vi "Main NR.vi"(8 "error in":errorcluster, 11 "cRIO NI 9205 Demo in":refnum<class "cRIO NI 9205 Demo.lvclass">) -> (0 "error out":errorcluster, 3 "cRIO NI 9205 Demo out":refnum<class "cRIO NI 9205 Demo.lvclass">)   [LabVIEW 2017, in "cRIO NI 9205 Demo.lvclass"]
doc: "The <b>Queued Message Handler</b> of the Worker that owns this VI."
uses:
  cRIO NI 9205 Demo.lvclass
  C:/Program Files (x86)/National Instruments/LabVIEW 2017/vi.lib/addons/_Workers/Library/Classes/Worker/Worker.lvclass
  cRIO NI 9205 Demo.lvclass/cRIO NI 9205 Demo.ctl
  Initialization Data.ctl
  TCP Client/TCP Client/rwr_Connect to Server.ctl
  Shared/TCP Data KEYS.ctl
  Shared/TCP Data Format.ctl
  TCP Client/TCP Client/rqp_Send String to Server.ctl
  <vilib>/addons/_Workers/Library/Classes/Message Queue/Message Queue.lvclass
  RT System Monitor/RT System Monitor.lvclass
  FPGA Read/FPGA Read.lvclass
  RT Watchdog/RT Watchdog.lvclass
  TCP Client/TCP Client/TCP Client.lvclass
panel:
  out "IP Address":string caption="Server IP Address"
  out "Server name":string caption="Server Name"
  out "Connected?":bool
  # "Server Connected"
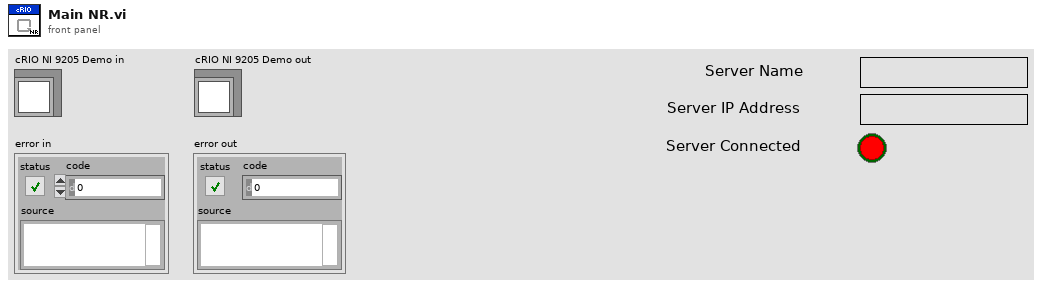
[diagram p1: front panel]
types:
  T1 = typedef "cRIO NI 9205 Demo.lvclass/Initialization Data.ctl" = cluster{"Client Name":string, "Server IP Address":string, "Server Port":u16, "Debugging Mode?":bool}
  T2 = typedef "TCP Client.lvlib/TCP Client.lvclass/rwr_Connect to Server.ctl" = cluster{"Client Name":string, "Server IP Address":string, "Server Port":u16}
  T3 = typedef "TCP Client.lvlib/TCP Client.lvclass/rqp_Send String to Server.ctl" = cluster{"String to Send":string}
  T4 = typedef "TCP Data Format.ctl" = cluster{"KEY":T5, "Data":string}
  T5 = typedef "TCP Data KEYS.ctl" = enum16{"RT System Monitor", "FPGA Data"}
  T6 = typedef "TCP Client.lvlib/TCP Client.lvclass/rsp_Connection Notify.ctl" = cluster{"Server Name":string, "IP Address":string, "Connected?":bool}
  T7 = typedef "RT System Monitor.lvclass/rsp_Receive System Properties.ctl" = cluster{"System Health Data":T8}
  T8 = typedef "System Health Data.ctl" = cluster{"CPUs":u32[][], "Memory":dbl[][], "Hard Drive Space Used (%)":dbl, "Primary Hard Drive Available (MB)":dbl, "Primary Hard Drive Capacity (MB)":u32, "Total Physical Memory (MB)":u32, "Total Virtual Memory (MB)":u32}
  T9 = typedef "FPGA Read.lvclass/rsp_Receive FPGA Data.ctl" = cluster{"FPGA Data":fxp<+/-,26,5>[]}
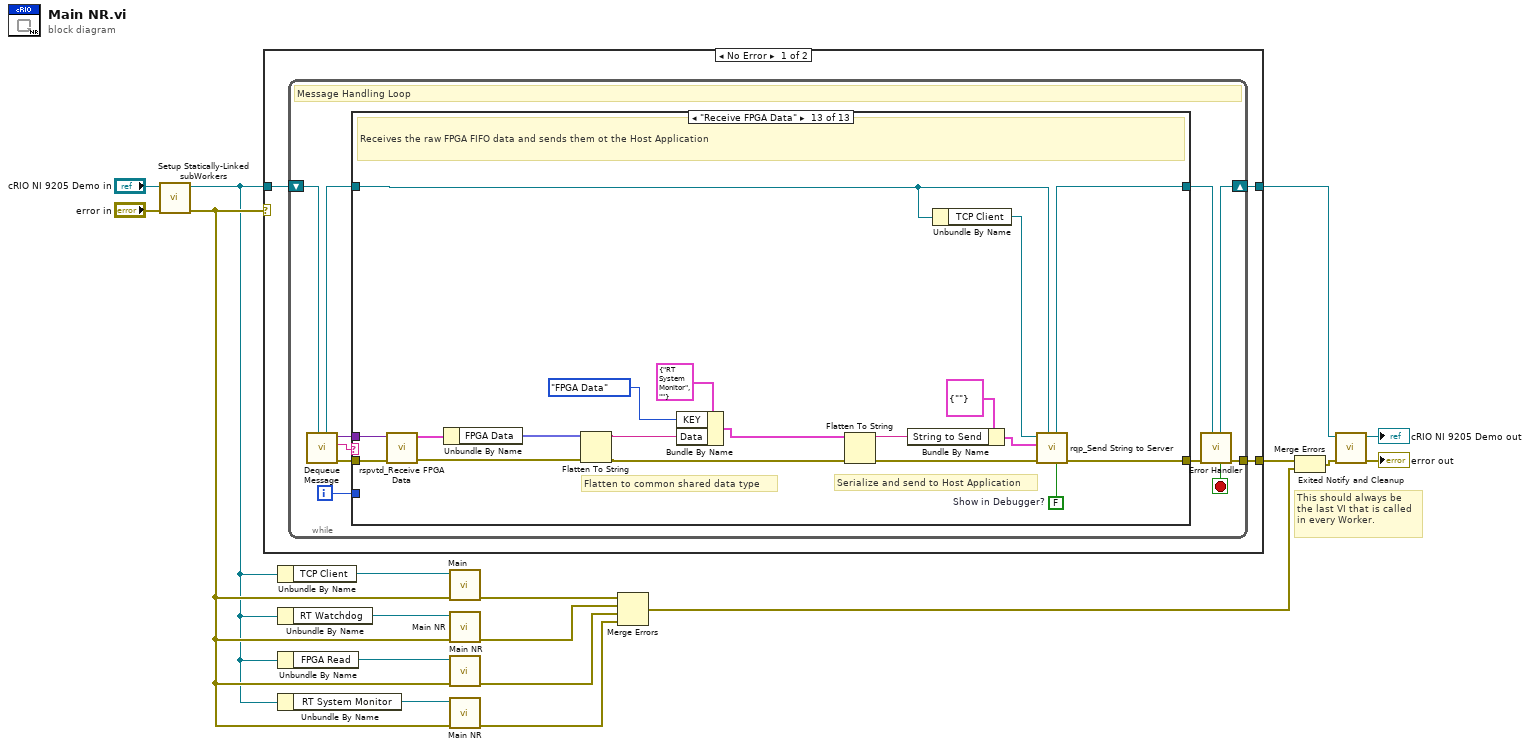
[diagram p0: block diagram]
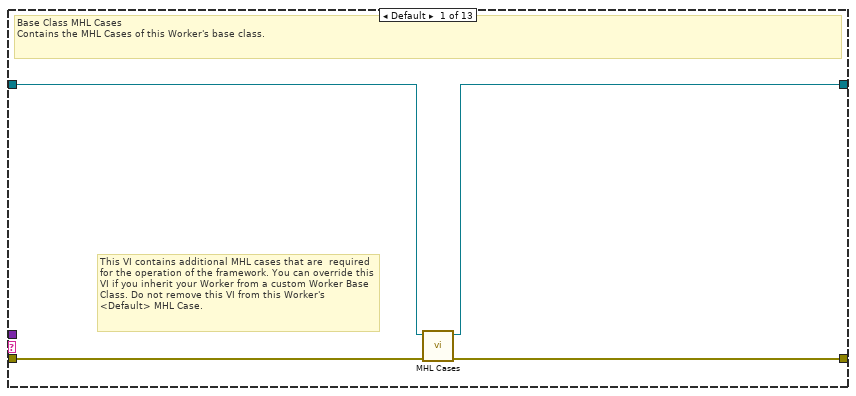
[diagram p2: hidden frame]
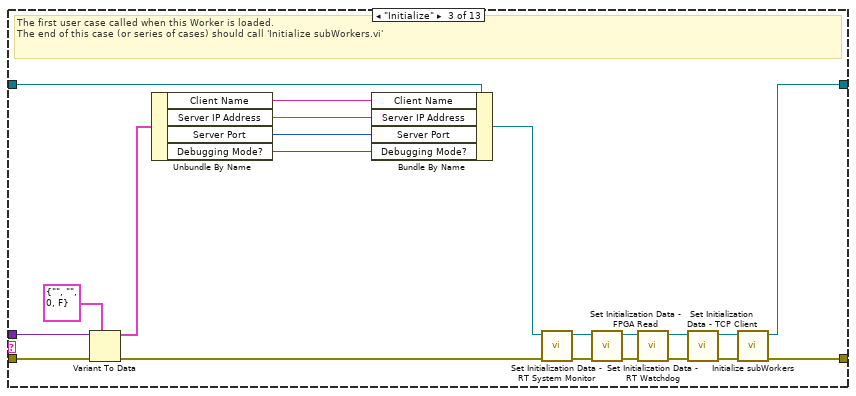
[diagram p4: hidden frame]
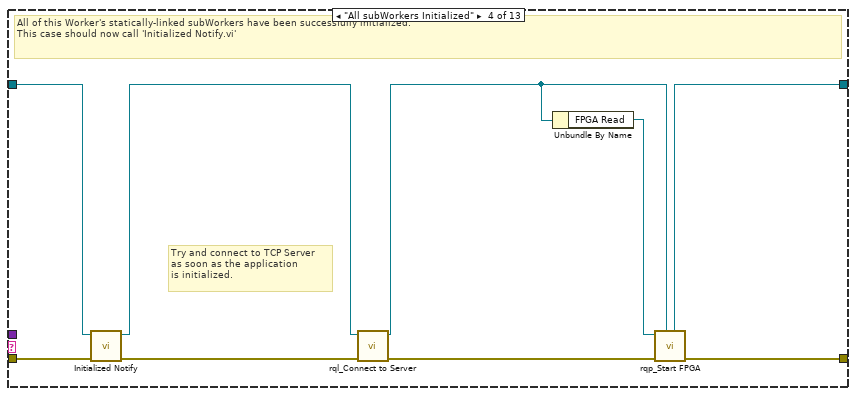
[diagram p5: hidden frame]
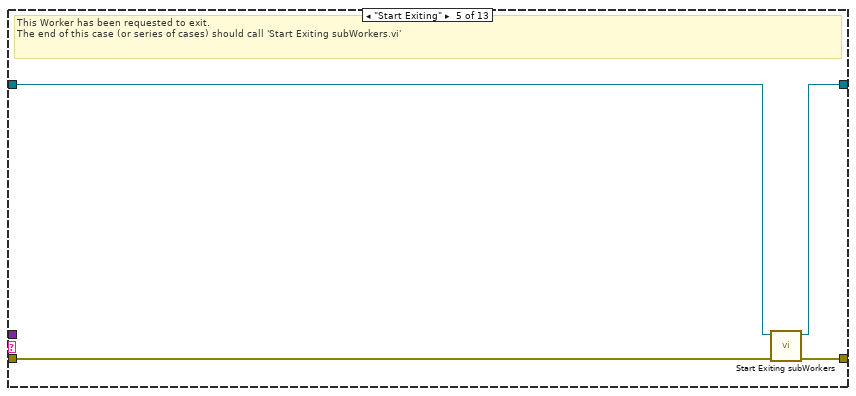
[diagram p6: hidden frame]
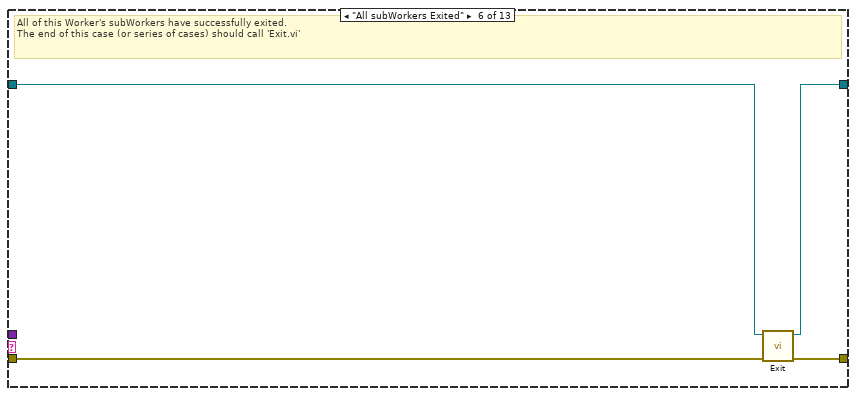
[diagram p7: hidden frame]
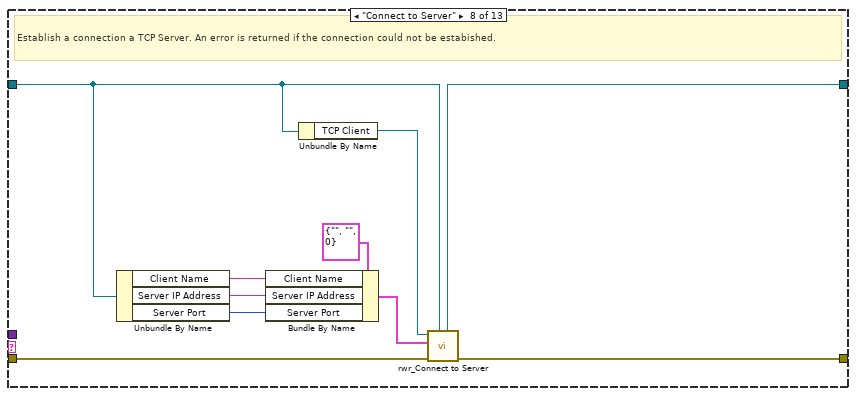
[diagram p9: hidden frame]
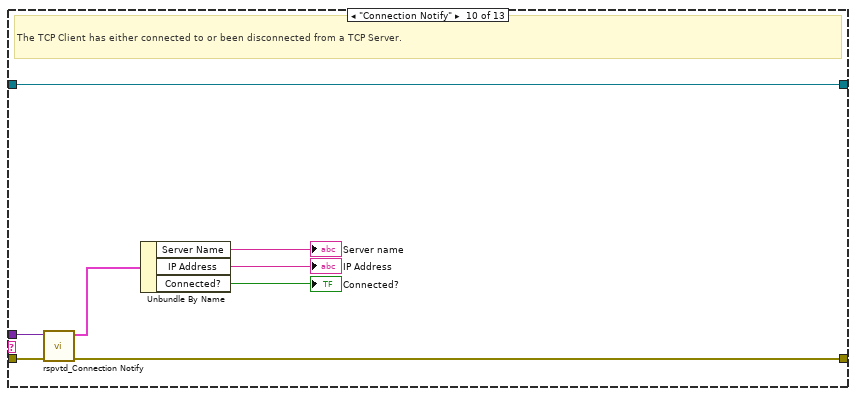
[diagram p11: hidden frame]
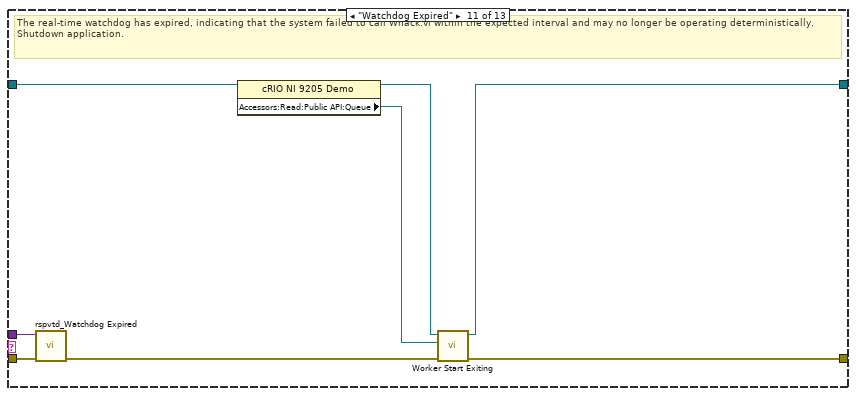
[diagram p12: hidden frame]
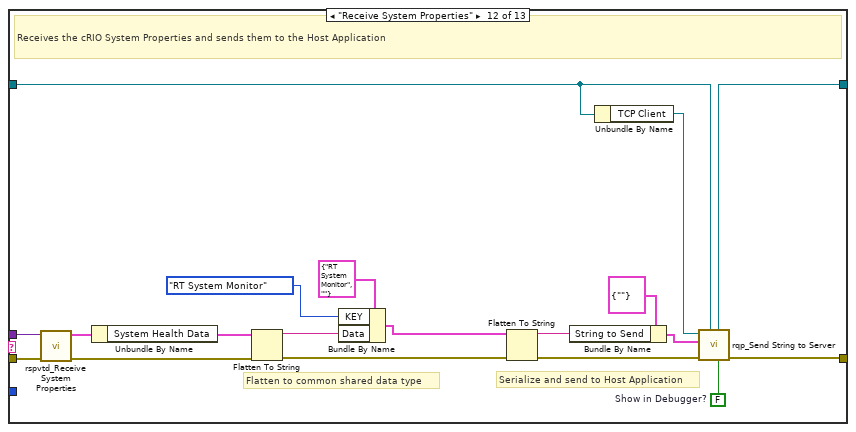
[diagram p13: hidden frame]
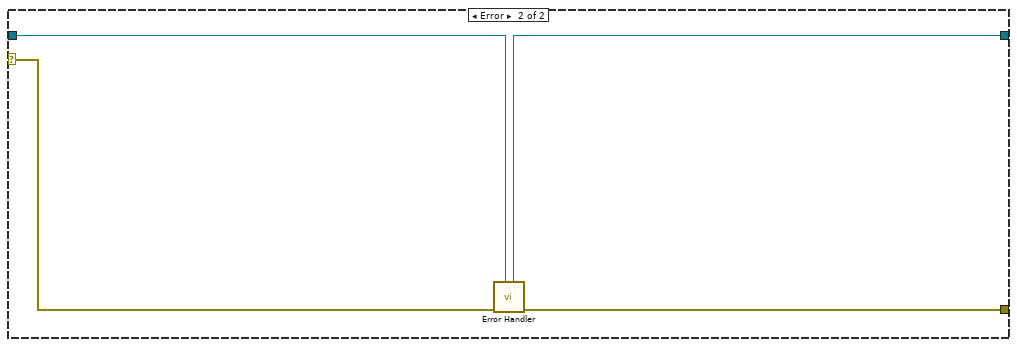
[diagram p14: hidden frame]
diagram:
  # "This should always be the last VI that is called in every Worker."
  n1 = call "Setup Statically-Linked subWorkers.vi"("error in"="error in", "cRIO NI 9205 Demo in"="cRIO NI 9205 Demo in") -> ("error out"=w12:errorcluster, "cRIO NI 9205 Demo out"=w10:refnum<class "cRIO NI 9205 Demo.lvclass">)  [unwired: 8 in]
  n2 = case shown="No Error" w12 {
    tunnel: w10 -> [w21 w146]
    tunnel: [w19 w147] -> w16
    tunnel: [w20 w145] -> w17
    selector: w12 -> [_ w148]
    frame No Error {
      n3 = while {
        shift-right: [w30] -> w20
        shift-left: w21 -> [w32]
        tunnel: [w31] -> w19
        i -> [w23]
        stop <- w24 stop-if-true
        # "Message Handling Loop"
        n4 = call-dynamic "Dequeue Message.vi"("Worker"=w32) -> ("error out"=w29:errorcluster, "Case out"=w25:string, "Data out"=w22:variant, "Worker out"=w27:refnum<class "cRIO NI 9205 Demo.lvclass">)  [unwired: 6 in, 1 out]
        n5 = case "Worker MHL Case Structure (DO NOT CHANGE LABEL NAME)" shown="\"Receive FPGA Data\"" w25 {
          tunnel: w29 -> [w36 w37 w57 w67 w69 w76 w78 w88 w90 w98 w106 w125 w144]
          tunnel: [w35 w37 w59 w63 w72 w75 w78 w87 w90 w96 w103 w114 w128] -> w28
          tunnel: w27 -> [w34 w38 w50 w68 w70 w74 w77 w82 w89 w97 w102 w113 w130]
          tunnel: [w33 w38 w58 w62 w71 w73 w77 w86 w89 w97 w101 w115 w129] -> w26
          tunnel: w23 -> [_ _ _ _ _ _ _ _ _ _ _ _ _]
          tunnel: w22 -> [_ _ w55 _ _ _ _ _ _ w95 w104 w124 w143]
          frame Default {
            # "This VI contains additional MHL cases that are  required for the operation of the framework. You can override this VI if you inherit your Worker from a custom Worker Base Class. Do not remove this VI from this Worker's <Default> MHL Case."
            # "Base Class MHL Cases\nContains the MHL Cases of this Worker's base class."
            n6 = call-dynamic "MHL Cases.vi"("error in"=w36, "Worker in"=w34) -> ("error out"=w35:errorcluster, "Worker out"=w33:refnum<class "cRIO NI 9205 Demo.lvclass">)  [unwired: 8 in]
          }
          frame "------------ FRAMEWORK CASES -----------" {
            # "Start of Workers Framework Cases"
          }
          frame "Initialize" {
            # "The first user case called when this Worker is loaded.\nThe end of this case (or series of cases) should call 'Initialize subWorkers.vi'"
            n7 = Variant To Data(error in=w57, type=T1 {"Client Name"="", "Server IP Address"="", "Server Port"=0, "Debugging Mode?"=FALSE} ("Initialization Data"), Variant=w55) -> (data=w53:T1, error out=w56:errorcluster)
            n8 = Unbundle By Name(w53) -> ("Client Name"=w49:string, "Server IP Address"=w48:string, "Server Port"=w47:u16, "Debugging Mode?"=w44:bool)
            n9 = Bundle By Name(cluster=w50, "Client Name"=w49, "Server IP Address"=w48, "Server Port"=w47, "Debugging Mode?"=w44) -> (w40:refnum<class "cRIO NI 9205 Demo.lvclass">)
            n10 = call "Set Initialization Data - RT System Monitor.vi"("error in"=w56, "cRIO NI 9205 Demo in"=w40) -> ("error out"=w41:errorcluster, "cRIO NI 9205 Demo out"=w39:refnum<class "cRIO NI 9205 Demo.lvclass">)  [unwired: 8 in]
            n11 = call "Set Initialization Data - FPGA Read.vi"("error in"=w41, "cRIO NI 9205 Demo in"=w39) -> ("error out"=w42:errorcluster, "cRIO NI 9205 Demo out"=w43:refnum<class "cRIO NI 9205 Demo.lvclass">)  [unwired: 8 in]
            n12 = call "Set Initialization Data - RT Watchdog.vi"("error in"=w42, "cRIO NI 9205 Demo in"=w43) -> ("error out"=w46:errorcluster, "cRIO NI 9205 Demo out"=w45:refnum<class "cRIO NI 9205 Demo.lvclass">)  [unwired: 8 in]
            n13 = call "Set Initialization Data - TCP Client.vi"("error in"=w46, "cRIO NI 9205 Demo in"=w45) -> ("error out"=w52:errorcluster, "cRIO NI 9205 Demo out"=w51:refnum<class "cRIO NI 9205 Demo.lvclass">)  [unwired: 8 in]
            n14 = call-dynamic "Initialize subWorkers.vi"("error in"=w52, "Worker"=w51) -> ("error out"=w59:errorcluster, "dup Worker out"=w58:refnum<class "cRIO NI 9205 Demo.lvclass">)  [unwired: 8 in]
          }
          frame "All subWorkers Initialized" {
            # "Try and connect to TCP Server\nas soon as the application\nis initialized."
            # "All of this Worker's statically-linked subWorkers have been successfully initialized.\nThis case should now call 'Initialized Notify.vi'"
            n15 = call-dynamic "Initialized Notify.vi"("error in"=w67, "Worker"=w68) -> ("error out"=w64:errorcluster, "dup Worker out"=w65:refnum<class "cRIO NI 9205 Demo.lvclass">)  [unwired: 8 in]
            n16 = call "rql_Connect to Server.vi"("error in"=w64, "cRIO NI 9205 Demo in"=w65) -> ("error out"=w66:errorcluster, "dup cRIO NI 9205 Demo out"=w61:refnum<class "cRIO NI 9205 Demo.lvclass">)  [unwired: 8 in]
            n17 = Unbundle By Name(w61) -> ("FPGA Read"=w60:refnum<class "FPGA Read.lvclass">)
            n18 = call "rqp_Start FPGA.vi"("Caller in"=w61, "error in"=w66, "FPGA Read in"=w60) -> ("error out"=w63:errorcluster, "dup Caller out"=w62:refnum<class "cRIO NI 9205 Demo.lvclass">)  [unwired: 6 in, 1 out]
          }
          frame "Start Exiting" {
            # "This Worker has been requested to exit. \nThe end of this case (or series of cases) should call 'Start Exiting subWorkers.vi'"
            n19 = call-dynamic "Start Exiting subWorkers.vi"("error_in"=w69, "Worker"=w70) -> ("error out"=w72:errorcluster, "dup Worker out"=w71:refnum<class "cRIO NI 9205 Demo.lvclass">)  [unwired: 8 in]
          }
          frame "All subWorkers Exited" {
            # "All of this Worker's subWorkers have successfully exited. \nThe end of this case (or series of cases) should call 'Exit.vi'"
            n20 = call-dynamic "Exit.vi"("error_in"=w76, "Worker"=w74) -> ("error out"=w75:errorcluster, "dup Worker out"=w73:refnum<class "cRIO NI 9205 Demo.lvclass">)  [unwired: 8 in]
          }
          frame "------------- LOCAL API CASES -------------" {
            # "Start of Workers Local API Cases"
          }
          frame "Connect to Server" {
            # "Establish a connection a TCP Server. An error is returned if the connection could not be estabished."
            n21 = Unbundle By Name(w82) -> ("Client Name"=w81:string, "Server IP Address"=w80:string, "Server Port"=w79:u16)
            n22 = Bundle By Name(cluster=T2 {"Client Name"="", "Server IP Address"="", "Server Port"=0} ("Connect to Server Data"), "Client Name"=w81, "Server IP Address"=w80, "Server Port"=w79) -> (w84:T2)
            n23 = Unbundle By Name(w82) -> ("TCP Client"=w83:refnum<class "TCP Client.lvclass">)
            n24 = call "rwr_Connect to Server.vi"("Caller in"=w82, "error in"=w88, "Data in"=w84, "TCP Client in"=w83) -> ("error out"=w87:errorcluster, "dup Caller out"=w86:refnum<class "cRIO NI 9205 Demo.lvclass">)  [unwired: 4 in, 2 out]
          }
          frame "------------- RESPONSE CASES --------------" {
            # "Start of Workers Response Cases"
          }
          frame "Connection Notify" {
            # "The TCP Client has either connected to or been disconnected from a TCP Server."
            n25 = call "rspvtd_Connection Notify.vi"("error in"=w98, "Data in"=w95) -> ("error out"=w96:errorcluster, "Data out"=w92:T6)  [unwired: 8 in]
            n26 = Unbundle By Name(w92) -> ("Server Name"=→"Server name":string, "IP Address"=→"IP Address":string, "Connected?"=→"Connected?":bool)
          }
          frame "Watchdog Expired" {
            # "The real-time watchdog has expired, indicating that the system failed to call Whack.vi within the expected interval and may no longer be operating deterministically. Shutdown application."
            n27 = call "rspvtd_Watchdog Expired.vi"("error in"=w106, "Data in"=w104) -> ("error out"=w105:errorcluster)  [unwired: 8 in, 1 out]
            n28 = property class="cRIO NI 9205 Demo"(reference=w102) -> (reference out=w100:refnum<class "cRIO NI 9205 Demo.lvclass">, "Accessors:Read:Public API:Queue"=w99:refnum<class "Message Queue.lvclass">)  [unwired: 1 in, 1 out]
            n29 = call-dynamic "Worker Start Exiting.vi"("error_in"=w105, "Message Queue"=w99, "Worker"=w100) -> ("error out"=w103:errorcluster, "dup Worker out"=w101:refnum<class "cRIO NI 9205 Demo.lvclass">)  [unwired: 7 in]
          }
          frame "Receive System Properties" {
            w122 = FALSE  # Show in Debugger?
            # "Flatten to common shared data type"
            # "Serialize and send to Host Application"
            # "Receives the cRIO System Properties and sends them to the Host Application"
            n30 = call "rspvtd_Receive System Properties.vi"("error in"=w125, "Data in"=w124) -> ("error out"=w117:errorcluster, "Data out"=w118:T7)  [unwired: 8 in]
            n31 = Unbundle By Name(w118) -> ("System Health Data"=w116:T8)
            n32 = Flatten To String(anything=w116, error in (no error)=w117) -> (data string=w121:string, error out=w120:errorcluster)  [unwired: 2 in, 1 out]
            n33 = Bundle By Name(cluster=T4 {"KEY"=enum."RT System Monitor", "Data"=""} ("TCP Data"), "KEY"=TCP_Data_KEYS."RT System Monitor", "Data"=w121) -> (w108:T4)
            n34 = Flatten To String(anything=w108, error in (no error)=w120) -> (data string=w107:string, error out=w109:errorcluster)  [unwired: 2 in, 1 out]
            n35 = Bundle By Name(cluster=T3 {"String to Send"=""} ("Data in"), "String to Send"=w107) -> (w110:T3)
            n36 = Unbundle By Name(w113) -> ("TCP Client"=w119:refnum<class "TCP Client.lvclass">)
            n37 = call "rqp_Send String to Server.vi"("Show in Debugger?"=w122, "Caller in"=w113, "error in"=w109, "Data in"=w110, "TCP Client in"=w119) -> ("error out"=w114:errorcluster, "dup Caller out"=w115:refnum<class "cRIO NI 9205 Demo.lvclass">)  [unwired: 4 in, 1 out]
          }
          frame "Receive FPGA Data" {
            w139 = FALSE  # Show in Debugger?
            # "Flatten to common shared data type"
            # "Serialize and send to Host Application"
            # "Receives the raw FPGA FIFO data and sends them ot the Host Application"
            n38 = call "rspvtd_Receive FPGA Data.vi"("error in"=w144, "Data in"=w143) -> ("error out"=w140:errorcluster, "Data out"=w142:T9)  [unwired: 8 in]
            n39 = Unbundle By Name(w142) -> ("FPGA Data"=w141:fxp<+/-,26,5>[])
            n40 = Flatten To String(anything=w141, error in (no error)=w140) -> (data string=w126:string, error out=w127:errorcluster)  [unwired: 2 in, 1 out]
            n41 = Bundle By Name(cluster=T4 {"KEY"=enum."RT System Monitor", "Data"=""} ("TCP Data"), "KEY"=TCP_Data_KEYS."FPGA Data", "Data"=w126) -> (w133:T4)
            n42 = Flatten To String(anything=w133, error in (no error)=w127) -> (data string=w132:string, error out=w134:errorcluster)  [unwired: 2 in, 1 out]
            n43 = Bundle By Name(cluster=T3 {"String to Send"=""} ("Data in"), "String to Send"=w132) -> (w135:T3)
            n44 = Unbundle By Name(w130) -> ("TCP Client"=w138:refnum<class "TCP Client.lvclass">)
            n45 = call "rqp_Send String to Server.vi"("Show in Debugger?"=w139, "Caller in"=w130, "error in"=w134, "Data in"=w135, "TCP Client in"=w138) -> ("error out"=w128:errorcluster, "dup Caller out"=w129:refnum<class "cRIO NI 9205 Demo.lvclass">)  [unwired: 4 in, 1 out]
          }
        }
        n46 = call-dynamic "Error Handler.vi"("Worker"=w26, "error_in"=w28) -> ("error out"=w31:errorcluster, "Stop Loop"=w24:bool, "Worker out"=w30:refnum<class "cRIO NI 9205 Demo.lvclass">)  [unwired: 7 in]
      }
    }
    frame Error {
      n47 = call-dynamic "Error Handler.vi"("Worker"=w146, "error_in"=w148) -> ("error out"=w147:errorcluster, "Worker out"=w145:refnum<class "cRIO NI 9205 Demo.lvclass">)  [unwired: 7 in, 1 out]
    }
  }
  n48 = Unbundle By Name(w10) -> ("TCP Client"=w7:refnum<class "TCP Client.lvclass">)
  n49 = Unbundle By Name(w10) -> ("RT Watchdog"=w5:refnum<class "RT Watchdog.lvclass">)
  n50 = Unbundle By Name(w10) -> ("FPGA Read"=w3:refnum<class "FPGA Read.lvclass">)
  n51 = Unbundle By Name(w10) -> ("RT System Monitor"=w1:refnum<class "RT System Monitor.lvclass">)
  n52 = call-dynamic "Main.vi"("error in"=w12, "TCP Client in"=w7) -> ("error out"=w9:errorcluster)  [unwired: 8 in, 1 out]
  n53 = call-dynamic "Main NR.vi"("error in"=w12, "RT Watchdog in"=w5) -> ("error out"=w6:errorcluster)  [unwired: 8 in, 1 out]
  n54 = call-dynamic "Main NR.vi"("error in"=w12, "FPGA Read in"=w3) -> ("error out"=w4:errorcluster)  [unwired: 8 in, 1 out]
  n55 = call-dynamic "Main NR.vi"("error in"=w12, "RT System Monitor in"=w1) -> ("error out"=w2:errorcluster)  [unwired: 8 in, 1 out]
  n56 = Merge Errors(w9, w6, w4, w2) -> (w8:errorcluster)
  n57 = Merge Errors(w16, w8) -> (w18:errorcluster)
  n58 = call-dynamic "Exited Notify and Cleanup.vi"("error_in"=w18, "Worker"=w17) -> ("error out"=→"error out":errorcluster, "dup Worker out"=→"cRIO NI 9205 Demo out":refnum<class "cRIO NI 9205 Demo.lvclass">)  [unwired: 8 in]
